vi "StringID to Num.vi"(10 "Driver Label":T3, 11 "Manipulator Label":T4) -> (2 "Driver Control Indexes":T1, 3 "Manipulator Control Indexes":T2)   [LabVIEW 2015]
uses:
  Common Code/Manipulator Control Label.ctl
  Common Code/Driver Control Label.ctl
  Common Code/Manipulator Control Indexes.ctl
  Common Code/Driver Control Indexes.ctl
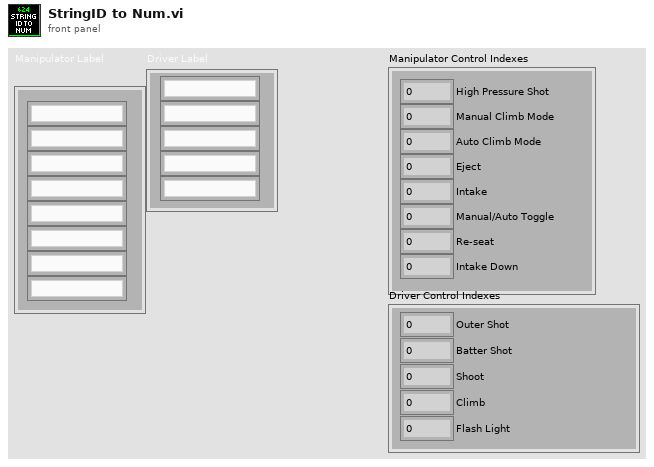
[diagram p1: front panel]
types:
  T1 = typedef "Driver Control Indexes.ctl" = cluster{"Outer Shot":dbl, "Batter Shot":dbl, "Shoot":dbl, "Climb":dbl, "Flash Light":dbl}
  T2 = typedef "Manipulator Control Indexes.ctl" = cluster{"High Pressure Shot":dbl, "Manual Climb Mode":dbl, "Auto Climb Mode":dbl, "Eject":dbl, "Intake":dbl, "Manual/Auto Toggle":dbl, "Re-seat":dbl, "Intake Down":dbl}
  T3 = typedef "Driver Control Label.ctl" = cluster{"Outer Shot":string, "Batter Shot":string, "Shoot":string, "Climb":string, "Flashlight":string}
  T4 = typedef "Manipulator Control Label.ctl" = cluster{"High Pressure Shot":string, "Manual Climb Mode":string, "Auto Climb Mode":string, "Eject":string, "Intake":string, "Manual/Auto Toggle":string, "Re-seat":string, "Intake Down":string}
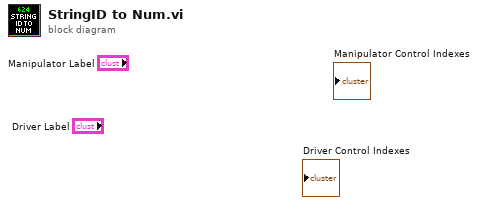
[diagram p0: block diagram]
diagram:
